vi "Read DispSnsr Obj.vi"(11 "DispSnsr Configuration in":refnum<class "DispSnsr Configuration.lvclass">) -> (2 "Hardware.lvlib:Displacement Sensor.lvlib:DispSnsr.lvclass":refnum<class "DispSnsr.lvclass">, 3 "DispSnsr Configuration out":refnum<class "DispSnsr Configuration.lvclass">)   [LabVIEW 2016, in "Hardware.lvlib" / "Displacement Sensor.lvlib" / "DispSnsr Configuration.lvclass"]
uses:
  <userlib>/Common Components/Hardware/Displacement Sensor/DispSnsr Config/DispSnsr Configuration.lvclass
  <userlib>/Common Components/Hardware/Displacement Sensor/DispSnsr/DispSnsr.lvclass
  <userlib>/Common Components/Hardware/Displacement Sensor/DispSnsr Config/DispSnsr Configuration.lvclass/DispSnsr Configuration.ctl
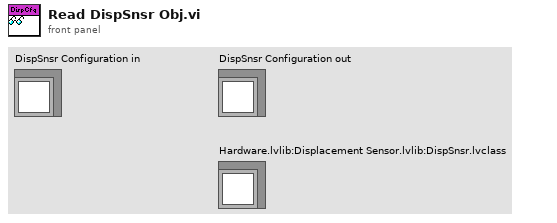
[diagram p1: front panel]
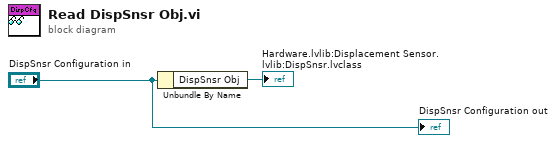
[diagram p0: block diagram]
diagram:
  n1 = Unbundle By Name("DispSnsr Configuration in") -> ("DispSnsr Obj"=→"Hardware.lvlib:Displacement Sensor.lvlib:DispSnsr.lvclass":refnum<class "DispSnsr.lvclass">)
  "DispSnsr Configuration out" <- "DispSnsr Configuration in"
